vi "cache tag indices.vi"(8 "error in":errorcluster, 9 "index cluster":variant, 10 "channel classification":T1, 11 "Temperature Chamber Model runtime in":refnum<class "Temperature Chamber Model runtime.lvclass">) -> (0 "error out":errorcluster, 3 "Temperature Chamber Model runtime out":refnum<class "Temperature Chamber Model runtime.lvclass">)   [LabVIEW 2013, in "Temperature Chamber Model runtime.lvclass"]
uses:
  Temperature Chamber Model runtime.lvclass
  configuration/parameter data indices.ctl
  configuration/Temperature Chamber Model configuration.lvclass
  configuration/result data indices.ctl
  <vilib>/NI/Tag Bus Module Framework/channel/channel classification.ctl
  <vilib>/NI/Tag Bus Module Framework/channel/TBM channel.lvclass
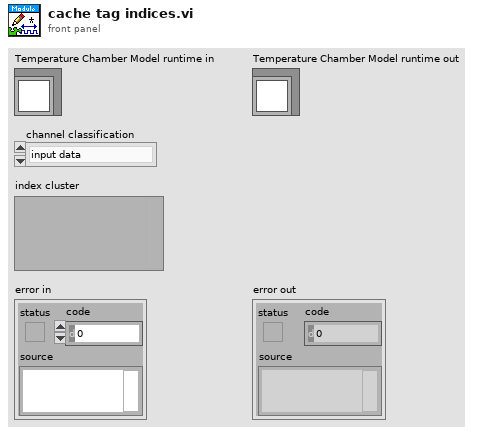
[diagram p1: front panel]
types:
  T1 = typedef "TBM channel.lvclass/channel classification.ctl" = enum16{"input data", "output data", "processing parameter", "processing result"}
  T2 = typedef "Temperature Chamber Model configuration.lvclass/parameter data indices.ctl" = cluster{"Double.Ambient Temperature":i32, "Double.Fan PWM":i32, "Double.Lamp PWM":i32}
  T3 = typedef "Temperature Chamber Model configuration.lvclass/result data indices.ctl" = cluster{"Double.Thermocouple Reading":i32}
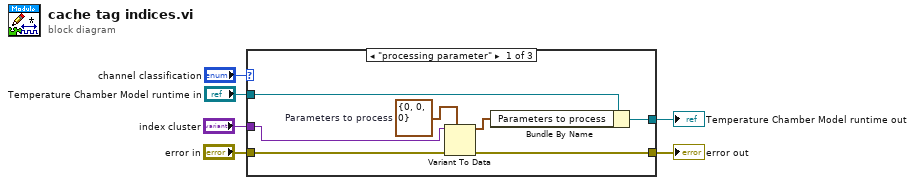
[diagram p0: block diagram]
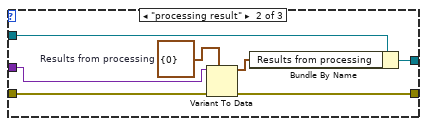
[diagram p2: hidden frame]
diagram:
  n1 = case shown="\"processing parameter\"" "channel classification" {
    tunnel: "index cluster" -> [w12 w19 _]
    tunnel: [w11 w18 w22] -> w4
    tunnel: "Temperature Chamber Model runtime in" -> [w10 w17 w22]
    tunnel: "error in" -> [w9 w16 w21]
    tunnel: [w8 w15 w21] -> w1
    frame "processing parameter" {
      w7 = T2 {"Double.Ambient Temperature"=0, "Double.Fan PWM"=0, "Double.Lamp PWM"=0}  # Parameters to process
      n2 = Variant To Data(error in=w9, type=w7, Variant=w12) -> (data=w13:T2, error out=w8:errorcluster)
      n3 = Bundle By Name(cluster=w10, "Parameters to process"=w13) -> (w11:refnum<class "Temperature Chamber Model runtime.lvclass">)
    }
    frame "processing result" {
      w14 = T3 {"Double.Thermocouple Reading"=0}  # Results from processing
      n4 = Variant To Data(error in=w16, type=w14, Variant=w19) -> (data=w20:T3, error out=w15:errorcluster)
      n5 = Bundle By Name(cluster=w17, "Results from processing"=w20) -> (w18:refnum<class "Temperature Chamber Model runtime.lvclass">)
    }
    frame Default {
    }
  }
  "error out" <- w1
  "Temperature Chamber Model runtime out" <- w4
